vi "Check_Out.vi"(7 "LabVIEW Web Service Request":refnum<class "Web Request.lvclass">) -> ()   [LabVIEW 2016]
uses:
  <vilib>/wsapi/Web Request.lvclass
  Device Info.ctl
  Inventory FGV Command.ctl
  Update Screen.ctl
panel:
  out "error out":errorcluster
  # "Use the Web Service Request input terminal to call the VIs on the Web Services palette. Do not remove it from the connector pane unless you don't need access to the palette."
  # "Each additional control wired to the connector pane will be available as an input in the URL. To include an indicator in terminal-mode output (the default setting), it must also be wired to the connector pane."
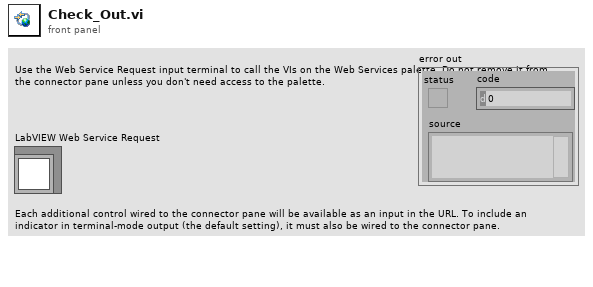
[diagram p1: front panel]
types:
  T1 = typedef "Update Screen.ctl" = cluster{"Time":string, "Item":string, "Name":string, "Action":string}
  T2 = typedef "Inventory FGV Command.ctl" = enum16{"Load Items", "Check Status", "Return Items", "Check Out Items", "Add New Item", "Get All Items", "Remove Item", "Search"}
  T3 = typedef "Device Info.ctl" = cluster{"Model Number":string, "Identifier":string, "Available?":bool, "Owner":string, "Owner Email":string, "Last Activity Date":string, "Loan Purpose":string, "Department":string, "Notes":string, "Serial Number":string}
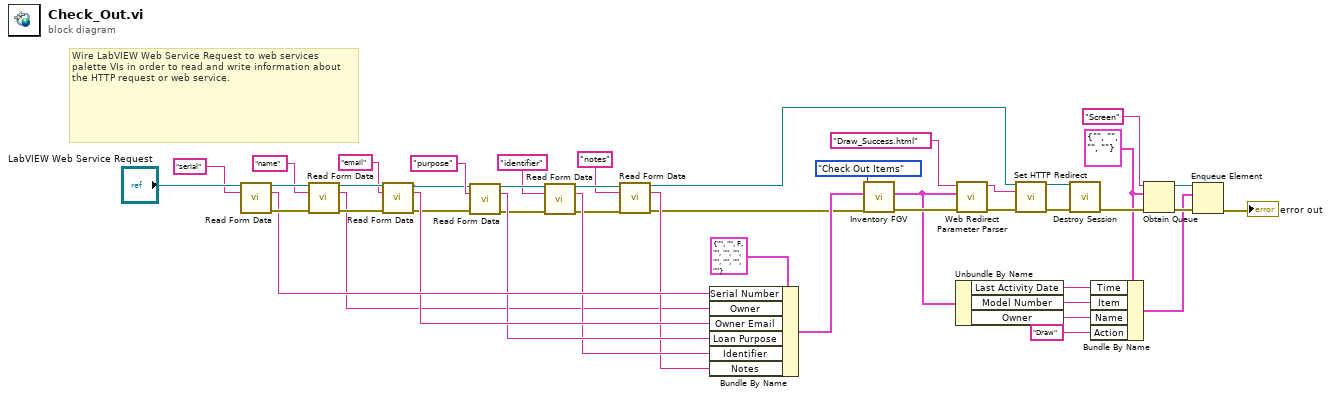
[diagram p0: block diagram]
diagram:
  w6 = T1 {"Time"="", "Item"="", "Name"="", "Action"=""}
  # "Wire LabVIEW Web Service Request to web services palette VIs in order to read and write information about the HTTP request or web service."
  n1 = call <vilib>:"Read Form Data.vi"("LabVIEW Web Service Request"="LabVIEW Web Service Request", "key"="serial") -> ("LabVIEW Web Service Request out"=w44:refnum<class "Web Request.lvclass">, "value"=w37:string, "error out"=w40:errorcluster)  [unwired: 10 in, 1 out]
  n2 = call <vilib>:"Read Form Data.vi"("LabVIEW Web Service Request"=w44, "key"="name", "error in (no error)"=w40) -> ("LabVIEW Web Service Request out"=w43:refnum<class "Web Request.lvclass">, "value"=w13:string, "error out"=w39:errorcluster)  [unwired: 9 in, 1 out]
  n3 = call <vilib>:"Read Form Data.vi"("LabVIEW Web Service Request"=w43, "key"="email", "error in (no error)"=w39) -> ("LabVIEW Web Service Request out"=w27:refnum<class "Web Request.lvclass">, "value"=w36:string, "error out"=w26:errorcluster)  [unwired: 9 in, 1 out]
  n4 = call <vilib>:"Read Form Data.vi"("LabVIEW Web Service Request"=w27, "key"="purpose", "error in (no error)"=w26) -> ("LabVIEW Web Service Request out"=w23:refnum<class "Web Request.lvclass">, "value"=w25:string, "error out"=w22:errorcluster)  [unwired: 9 in, 1 out]
  n5 = call <vilib>:"Read Form Data.vi"("LabVIEW Web Service Request"=w23, "key"="identifier", "error in (no error)"=w22) -> ("LabVIEW Web Service Request out"=w19:refnum<class "Web Request.lvclass">, "value"=w20:string, "error out"=w18:errorcluster)  [unwired: 9 in, 1 out]
  n6 = call <vilib>:"Read Form Data.vi"("LabVIEW Web Service Request"=w19, "key"="notes", "error in (no error)"=w18) -> ("LabVIEW Web Service Request out"=w15:refnum<class "Web Request.lvclass">, "value"=w16:string, "error out"=w14:errorcluster)  [unwired: 9 in, 1 out]
  n7 = Bundle By Name(cluster=T3 {"Model Number"="", "Identifier"="", "Available?"=FALSE, "Owner"="", "Owner Email"="", "Last Activity Date"="", "Loan Purpose"="", "Department"="", "Notes"="", "Serial Number"=""} ("Device"), "Serial Number"=w37, "Owner"=w13, "Owner Email"=w36, "Loan Purpose"=w25, "Identifier"=w20, "Notes"=w16) -> (w35:T3)
  n8 = call "Inventory FGV.vi"("error in"=w14, "Device Info"=w35, "Command"=Inventory_FGV_Command."Check Out Items") -> ("error out"=w32:errorcluster, "Device Info Out"=w12:T3)  [unwired: 5 in, 1 out]
  n9 = Unbundle By Name(w12) -> ("Last Activity Date"=w5:string, "Model Number"=w4:string, "Owner"=w3:string)
  n10 = call "Web Redirect Parameter Parser.vi"("redirect URL"="Draw_Success.html", "Device"=w12, "error in (no error)"=w32) -> ("Output String"=w29:string, "error out"=w31:errorcluster)  [unwired: 6 in]
  n11 = call <vilib>:"Set HTTP Redirect.vi"("LabVIEW Web Service Request"=w15, "redirect URL"=w29, "error in (no error)"=w31) -> ("LabVIEW Web Service Request out"=w34:refnum<class "Web Request.lvclass">, "error out"=w33:errorcluster)  [unwired: 11 in]
  n12 = call <vilib>:"Destroy Session.vi"("LabVIEW Web Service Request"=w34, "error in (no error)"=w33) -> ("error out"=w10:errorcluster)  [unwired: 12 in, 1 out]
  n13 = Bundle By Name(cluster=w6, "Time"=w5, "Item"=w4, "Name"=w3, "Action"="Draw") -> (w1:T1)
  n14 = Obtain Queue(name (unnamed)="Screen", element data type=w6, error in (no error)=w10) -> (queue out=w7:refnum<queue>, error out=w9:errorcluster)  [unwired: 2 in, 1 out]
  n15 = Enqueue Element(queue=w7, element=w1, error in (no error)=w9) -> (error out=→"error out":errorcluster)  [unwired: 1 in, 2 out]
